vi "mxwScript_API_XMLConnectToArrayOnConPane.vi"(6 "connection type":T1=enum."Recommended", 8 "error in (no error)":errorcluster, 9 "connectorPaneTerminal":u32, 10 "arrayName":string, 11 "arrayElementName":string) -> (0 "error out":errorcluster, 3 "encoded connectorPaneName":string)   [LabVIEW 2017]
doc: "Create encoded \"connectorPaneName\" for dynamically adding to a cluster connected to a specific connector pane terminal. The cluster is created if it does not exist using <B>clusterName</B>. If the cluster already exists, <B>clusterName</B> is ignored."
uses:
  codeGenAPISupport.llb/cgAPI_mxwScript_ConnPaneConnectionType.ctl
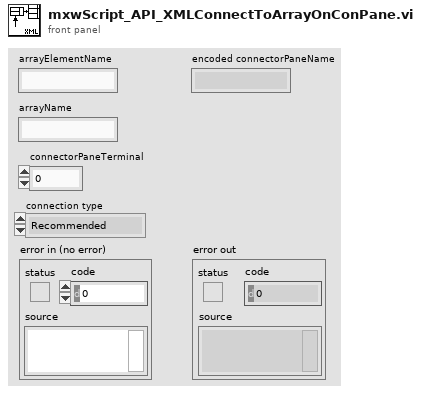
[diagram p1: front panel]
types:
  T1 = typedef "cgAPI_mxwScript_ConnPaneConnectionType.ctl" = enum16{"Invalid Wire Rule", "Required", "Recommended", "Optional", "Dynamic Dispatch"}
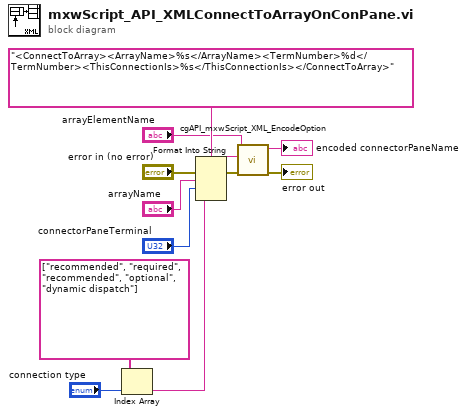
[diagram p0: block diagram]
diagram:
  n1 = Index Array(array=string[] ["recommended", "required", "recommended", "optional", "dynamic dispatch"], index="connection type") -> (element=w2:string)
  n2 = Format Into String(format string="<ConnectToArray><ArrayName>%s</ArrayName><TermNumber>%d</TermNumber><ThisConnectionIs>%s</ThisConnectionIs></ConnectToArray>" ("control name"), error in="error in (no error)", "arrayName", "connectorPaneTerminal", w2) -> (resulting string=w8:string, error out=w10:errorcluster)  [unwired: 1 in]
  n3 = call "cgAPI_mxwScript_XML_EncodeOption.vi"("error in (no error)"=w10, "otherXML"=w8, "normalTextString"="arrayElementName") -> ("error out"=→"error out":errorcluster, "encodedString"=→"encoded connectorPaneName":string)  [unwired: 7 out]
